vi "Day 4 Task 2.vi"() -> ()   [LabVIEW 2018]
uses:
  <userlib>/_OpenG.lib/array/array.llb/Search 1D Array (I32)__ogtk.vi
  <userlib>/_OpenG.lib/array/array.llb/Conditional Auto-Indexing Tunnel (I32)__ogtk.vi
panel:
  out "all cards won?":bool
  out "final score":i32
  out "number callled":i32
  out "someone won?":bool
  out "card that won":i32
  out "cards":i32[][][](array[numeric])
  out "numbers called out":i32[](array[numeric])
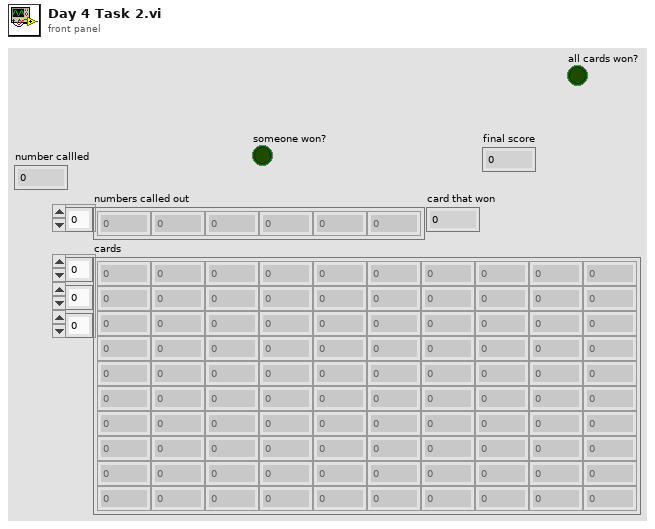
[diagram p1: front panel]
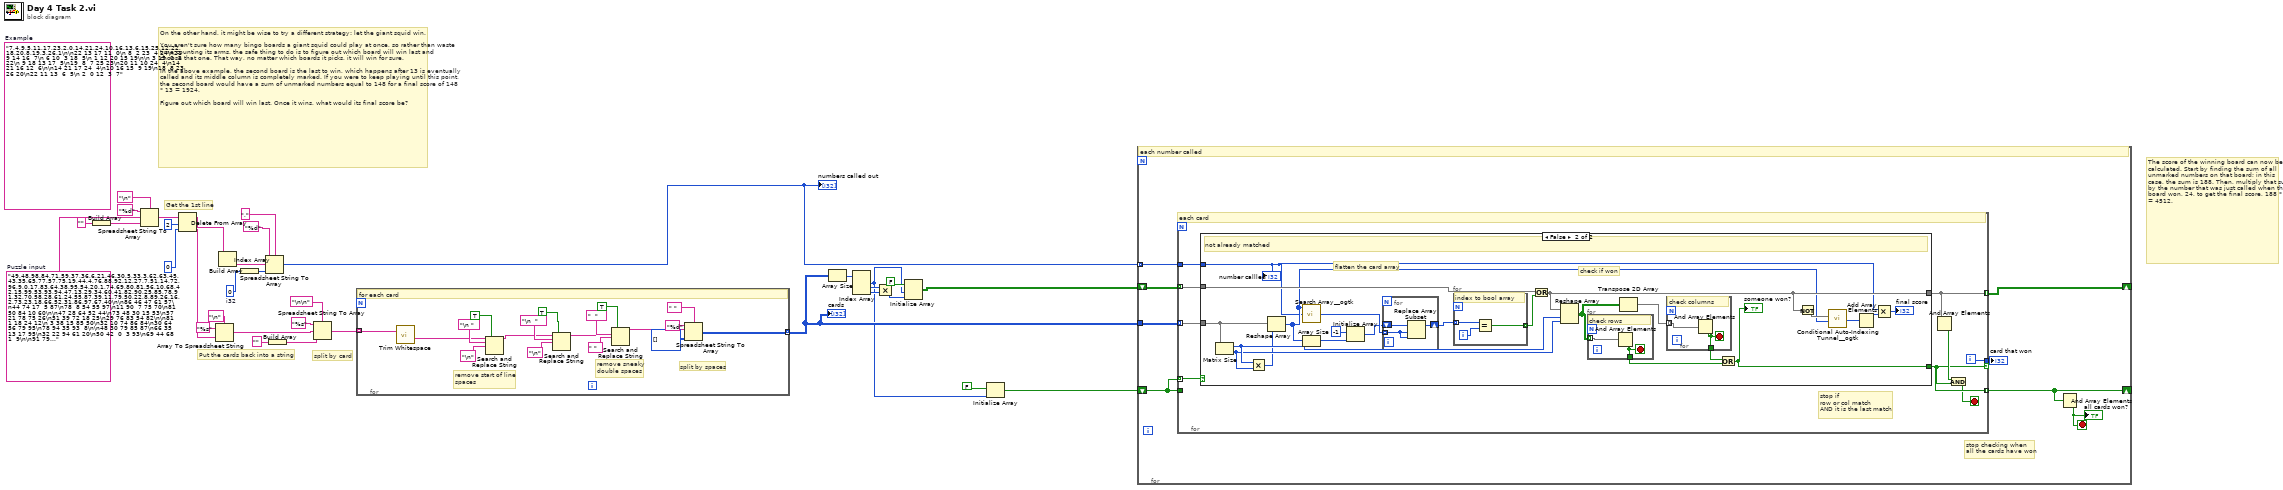
[diagram p0: block diagram]
diagram:
  w1 = "49,48,98,84,71,59,37,36,6,21,46,30,5,33,3,62,63,45,43,35,65,77,57,75,19,44,4,76,88,92,12,27,7,51,14,72,96,9,0,17,83,64,38,95,54,20,1,74,69,80,81,56,10,68,42,15,99,53,93,94,47,13,29,34,60,41,82,90,25,85,78,91,32,70,58,28,61,24,55,87,39,11,79,50,22,8,89,26,16,2,73,23,18,66,52,31,86,97,67,40\n\n86 46 47 61 57\n44 74 17  5 87\n78  8 54 55 97\n11 90  7 75 70\n81 50 84 10 60\n\n47 28 64 52 44\n73 48 30 15 53\n57 21 78 75 26\n51 39 72 18 25\n29 76 83 54 82\n\n81  1 18 24 12\n 3 38 15 85 50\n32 10 74 86 84\n30 64 56 79 95\n78 94 35 93  8\n\n48 30 79 85 87\n66 35 13 17 95\n32 22 94 61 20\n50 42  0  3 93\n69 44 68  1  9\n\n91 79 93 41 33\n98 51 39  9 10\n24 70 99  2 11\n32 13 21  6 68\n40 27 48 89  7\n\n40 29 34  1 23\n79 36 75 57 95\n61 50  4 21 48\n54  0 81 98 72\n24 30 15 31 52\n\n18 68 17 25 34\n97 36 77  6 30\n79 72 38 94 60\n54 45 16 67 12\n58 31 57 71 92\n\n40 58 80 86 85\n91 57 51 23 10\n61 78  4 36 66\n24 41 88 25 99\n15 68 12 55 75\n\n82 99 17  5 76\n65 42 73 78 61\n34 62 14 23 68\n 9 79 72 45  0\n43 96 11 13 10\n\n98 47 90 14 12\n80 63 35 42 11\n27 66  1  9 32\n17 85 61 71 68\n 6 29  7 94 67\n\n38 35 70 18 59\n62 54 84 10 27\n60 92 90 64 86\n25 99 49 43  4\n23 50 39 16 40\n\n72  1 73  8 33\n86 65 99 49 66\n56 79 23 41 46\n 4 48 43 55 93\n98 63 47 37 30\n\n33 96 72 93 99\n30 12 56 46 65\n39 40 59 94 50\n 0  8 67 27 47\n53 57 24 77 42\n\n 9 57  8 28 12\n90 81 21 25 51\n88 18 78  3 64\n20 87 97 45 85\n92 40 52 29 17\n\n99 89 15 54 32\n93 81 36 14 91\n86  7 67 18 92\n65 21 55 38  8\n12 88 27 90 94\n\n96  0  6 91 44\n28 60 10 70 75\n69 37 51 21 87\n93 59 14 53 15\n64 66  9 50 27\n\n33 46 38  2 41\n24 51 50 72 57\n42 85 99 97 56\n35 69 12 86 73\n 4 47 34 80 17\n\n70 28 77 73 53\n67 94 83 79 82\n89  9 96 48 17\n47 86 88 12  3\n55 39 98 14 90\n\n64 82 85 45 10\n27  5 12 72 40\n52 31 25 79 65\n 6 26  3 43 57\n89 49 36 59 35\n\n70  0 58 98 65\n54 93 75 14 26\n28 69 17 29 78\n46 22 47 85 87\n44 38 10 11 63\n\n18 52 66 42 58\n99 78 44 28 73\n24 71  5 14 82\n77 35 45 76 19\n70 20  0 43 48\n\n42 82 85 87 51\n40 49 93 95 74\n25 79 37 67 55\n26 27 90 47 22\n38 50 33 10 75\n\n15 99 60 28 79\n94 42 63 20 57\n44 55 96 67 53\n64  3 29 61 33\n51 12 39 97 30\n\n 7 95 28 39 76\n87 31 23 47 75\n88 10 78 24 20\n30 81 22 51 62\n53 93 55 38  0\n\n12 99  2 89 17\n30 23 92 66 10\n39 60 74 82 15\n 1 28 49  0 29\n90 55  9 69 83\n\n79 44 70 59 88\n90  8 81 23  5\n40 67 66 55 17\n95 61 75 48 91\n98 71 24 38 29\n\n95 28  8 76 13\n86 21 48  3  6\n34 47 31 50  2\n52 40 77 60 61\n 0 88 87 23 25\n\n63 70 34 91 17\n98 49  8  2 14\n25 22 92 65 18\n78 61 97 73 20\n57 83 16  7 68\n\n43 23 70 39 16\n 0 60 76  7 58\n89 40 38 17  5\n86 50 10 77 37\n26 65 25 69 92\n\n34 71 92 19 80\n93  6 24 42 45\n96  9 50 85 21\n36 49 13 25 17\n20 98 74 70 57\n\n25 96 65 77 30\n22 34 41 36 91\n62 18 61 15 19\n42 74 86 58 97\n87 31 53  8 52\n\n40 37 15 53 91\n14 11 35 49 55\n73 32 83 66 87\n98 31 70 58 88\n 7 61  8 76 16\n\n27 94 87 57 80\n54 35 40 59 72\n88 84 70 98 92\n37 52 45  7 16\n 0 30 12 22 41\n\n44 65 68 14 70\n 5 35 17 90  7\n56 89 48 84 32\n73 69 74 51 72\n24 10 94 78 60\n\n81 15  3 42 90\n54 52 74 84 71\n97 78 20  9  2\n59 66  1 91 87\n70 56 93 47 37\n\n93 36 19 69 94\n17 20 48 58 52\n85 57 90 42 14\n16 92  4 49 65\n22  9  2 24 44\n\n47 99 13 31 62\n81 58 88 91 94\n29 11 96 95  1\n14 20 82 34 37\n84 39 76 41 22\n\n 1 74 21  2 67\n38 79 96 26 88\n19 17 94 71 52\n31 28 69  8 51\n41 77 45 95 82\n\n24  9 94 69 65\n97 84 85 53  5\n92 11 61 77  8\n21 75 33 57 63\n43 68 55 52 93\n\n27 21  8 75 73\n 4 53 23 56 47\n28 94 50 80 19\n89 58 24 12 13\n60  5 99 96  9\n\n31 43 59 65 33\n51 32 14 58  4\n11 41 70 78 12\n 1 25 57 80 49\n91 66  0 27 17\n\n64 67 37 24 35\n 4 22 54 75 21\n19 91  9 52 83\n20 68 53 12  0\n28 76 51 49 89\n\n67 89 14 54 81\n 0 59 51 63 56\n85 88 95  7 36\n40 27 47 86 19\n52 92 22 16 30\n\n75 25 39  9 19\n59 92 24  6 22\n79 73 34 66 49\n16 89 56 76 55\n 5 45  4 46 62\n\n71 44 63 97 47\n27 61 70 52 46\n19 80 21 68 65\n28 45 84 14 94\n38 73 66 78 92\n\n47 45 41 96 54\n38 14 62 55 91\n 2 11 97 12 51\n36 49  3 95 76\n 5 75  7 94 87\n\n70 24 93 96 86\n49 51 73 50 83\n97  0 57 13  9\n99 46 22 67 39\n56 21 29 52 27\n\n42 82 80 65 19\n78 41 56 83 75\n51 72 10  1 33\n84 63 21 87 86\n77 64 31 68  6\n\n60 50 31  5 58\n83  9 87 98 13\n 4 35 24 33 88\n54 59 71 64  3\n16 57 48 15 86\n\n45 29 81 25 14\n13 21 79 90  0\n88 38 56 11 15\n47  2 40 35 75\n91 28 48 32 98\n\n87 58 78 65 69\n89 35 45 26 13\n28 61 15  3 44\n64 57 92 93 50\n90 39  4 70  9\n\n16 35 41 40 81\n48 92 94 83 79\n54 50 62  8 53\n14  5 85 68 22\n42 26 33 23 93\n\n 7 13 82 89 49\n43 21 79 38 56\n 6 31 90 58 81\n39 47 77 30 54\n23 41 86 19  8\n\n69 20 95 33 63\n64 34  4 79 36\n13 21 78 56  6\n35 44 85 27 76\n75 15 14 52 39\n\n42 71 73  1 45\n66 75  7 40 54\n91 83 65 53 20\n34 97 88  5 61\n63 82 50 74 38\n\n62 89 40 70 91\n84 12 19 96 79\n72 15 35 23 14\n 4 69  0 55 17\n85 90 20 28 13\n\n27 93 23  1 38\n67 28 62  9 96\n31 35 47 44 88\n78 57 53  5 69\n91 15 82 75 61\n\n17 44 85 92 94\n 0 67  5 50 64\n66 65 98 58 56\n62  4 57 99 34\n83 43 76 12 69\n\n 0 28 13 68 86\n84 24 50 32 40\n25 71 72 96 94\n89  1 64 81 23\n97 66  5 15 91\n\n59 67 79 84 44\n74 61 81 20 68\n24 92 55 99 11\n76 60 97 43 66\n31 30 89 45 53\n\n 1 97 15 34 85\n45 59 54 66 24\n53 36 51 58 27\n84 83 71  5 95\n70  6 65 79 13\n\n84 86  0 25  2\n 1 59 92 39 56\n17  7 88 78 24\n51 87 89 44 31\n54 63 50 18 36\n\n98 86 30 70 12\n11 52 49 39 14\n16 35 56 87 72\n85 65 93 92 60\n20 43 77 41 79\n\n50 31 71 78 21\n70 94 99 35 29\n56 58 27 65 28\n45 36 47 69 98\n 5 48 61 19 93\n\n64 65 86 14 53\n 7 43 75 39 38\n20 59 80 88 54\n12 32 66 34 87\n29 15 25 19 45\n\n88 20 42  5 32\n56  8 80 15 98\n36 99 35 27 16\n92 66 75 91 10\n81 96 65  0 57\n\n29 78  8 76 41\n99 18 60 90 47\n50 51 40  2 31\n38 70 25 52 39\n26 35 84  6 80\n\n 6 68 56 15 53\n99 60 69 25  7\n65 35  9 11 66\n92 85 48 40 97\n63 59 57 17 55\n\n46 95 75 99 21\n50 24 64 35 63\n93 39  3 67 82\n41 42 84 15 55\n79 81 97 60 17\n\n33 14 60 42 40\n76 73 56 71 88\n91 41 83 74 16\n57 85 35 44 47\n99 59 46 12 45\n\n53 83 54 21 68\n79 97 85  0 67\n41 90 48 95  3\n96 70 65 22 25\n60 77 33 15 28\n\n17 12  5 51 15\n75 92 72 16 65\n59 85 29 23 57\n14 53 97 68 84\n 1 93 49 38 28\n\n27 40 24 12 57\n84 13  9 43 31\n70 23 51 94 34\n 1 80 91 16 29\n99 75 49 52 54\n\n52 85 23 72 40\n 6 88 16 41 67\n53 94  8 32 33\n75 62 24 13 64\n65  0 60 86 47\n\n 5 28 27 15 41\n19 77 38 83 45\n32 70 78 26 90\n82 80 85 22 84\n59 73 24  9 63\n\n29 58 28 82 13\n78 55 63 43 51\n19 33 90 91 48\n93  7 35 22 71\n40 95 38 24 46\n\n38 30 13 16 74\n69 68 42  6  4\n62 82 29 79  1\n61  7 15 25 85\n 5 66 45 43 90\n\n19 65 12 91 34\n17  6 30 32 64\n37 53  4 35 62\n41 22 13 11 25\n60 27 93 76 51\n\n 3 92 25 88 14\n40 30 55 10 37\n19 94 56 34 74\n75 87 80 54 83\n 2 20 70 45 16\n\n52 93 87 60 11\n82 66 88 59 95\n58 31 49 33 28\n77 39 43  9 51\n20 80 98 47 16\n\n35 48 47 11 82\n 8 36 54 20 40\n90 95 85  4 66\n22 75 64 81 10\n27 62 89 30 12\n\n75 40 11 63 19\n 4 43  6 93 48\n85 58 82 66 52\n32 28  0 14 20\n78 61 83 95 87\n\n57 79 16 37 33\n20 17 27 38 63\n35 77 60 97 34\n22 78 72 43 26\n29 12  9 46 54\n\n26 94 37 57  1\n49  6 65 80 55\n46 38 33 89 99\n42 18 86 97 98\n45 76 41  9 12\n\n83 70 31 61 30\n16 78 84 12 18\n15 65 62 55 98\n 6 21 80 41 69\n25  2 24 10 79\n\n98 75  5 66 37\n90  7 26 61 15\n48 70 20 60 41\n23 58 82 22 74\n80  8 51 67 55\n\n84 86 77 97 28\n37 87  2 93  5\n16 64 35 61 27\n 8  3 36 10 73\n31 65 94 63 13\n\n91  9 64 67 19\n56 35 11 62 28\n 0 65 59 72 45\n34 24 51 26 80\n93 50 58 53 27\n\n27 54 77 57 94\n60 46 55 74 62\n16  9 19 48  6\n69  1 26 78  2\n45 75 41 25 90\n\n45 83 97 81 95\n26 64 40 94  7\n57 28 86  8 36\n98 92 16 13 20\n99 79 50 65 51\n\n38  6 96 71 10\n51 55  2 44 74\n31 61 98 72 73\n79 54 91 34 62\n88 17 46 45 43\n\n17 18 39 59 26\n45 40 91 47 74\n46 97 94 12 79\n61  7  8 56 50\n 0 77 20 57  9\n\n74  4 65  2 23\n45 56 90 94 96\n80 71 69 86 85\n19 78 35 47 98\n51 73  6 33 14\n\n 8 60 40  2 37\n10 68 44 50 73\n69 26  6 52 93\n33 65 46 24 11\n71 59 15 28 84\n\n57 65 70 98 68\n80  3 13 39 20\n11 71 47 78 42\n31 61 72 86  9\n53 43 87 28 77\n\n67 32 59 34 77\n29 23 80 27 62\n81 97 46 14 42\n19 47 44 85 24\n53  9 71 37  1\n\n83 13 27 41  9\n95 62 65 86 63\n 0 17 33 11 76\n45 64 39 71 55\n84 52 21 59 20\n\n63 45 55 80  3\n14 73 47 96 10\n82 26 85  0 11\n53  6 28 57 60\n49 99 18 50 71\n\n30 67 16 22 84\n81  4 34 61 65\n57 69 51 94 58\n 6 89 37 75 47\n19 14 97  2 86\n\n64 83  1 66 70\n30 82 96  3 67\n79 11 22 95 14\n87 60  4 15 26\n84 69 99 19 74"  # Puzzle input
  w13 = 0  # i32
  (unwired) "7,4,9,5,11,17,23,2,0,14,21,24,10,16,13,6,15,25,12,22,18,20,8,19,3,26,1\n\n22 13 17 11  0\n 8  2 23  4 24\n21  9 14 16  7\n 6 10  3 18  5\n 1 12 20 15 19\n\n 3 15  0  2 22\n 9 18 13 17  5\n19  8  7 25 23\n20 11 10 24  4\n14 21 16 12  6\n\n14 21 17 24  4\n10 16 15  9 19\n18  8 23 26 20\n22 11 13  6  5\n 2  0 12  3  7"  # Example
  # "On the other hand, it might be wise to try a different strategy: let the giant squid win.\n\nYou aren't sure how many bingo boards a giant squid could play at once, so rather than waste time counting its arms, the safe thing to do is to figure out which board will win last and choose that one. That way, no matter which boards it picks, it will win for sure.\n\nIn the above example, the second board is the last to win, which happens after 13 is eventually called and its middle column is completely marked. If you were to keep playing until this point, the second board would have a sum of unmarked numbers equal to 148 for a final score of 148 * 13 = 1924.\n\nFigure out which board will win last. Once it wins, what would its final score be?"
  # "The score of the winning board can now be calculated. Start by finding the sum of all unmarked numbers on that board; in this case, the sum is 188. Then, multiply that sum by the number that was just called when the board won, 24, to get the final score, 188 * 24 = 4512."
  # "split by card"
  # "Put the cards back into a string"
  # "Get the 1st line"
  n1 = Build Array("") -> (w31:string[])
  n2 = Spreadsheet String To Array(delimiter (Tab)="\n", format string="%d", spreadsheet string=w1, array type (2D Dbl)=w31) -> (array=w29:string[])
  n3 = Delete From Array(array=w29, length=2, index=0) -> (deleted portion=w24:string[], array with subset deleted=w21:string[])
  n4 = Array To Spreadsheet String(delimiter (Tab)="\n", array=w21, 3:"%s" ("format string")) -> (spreadsheet string=w19:string)
  n5 = Index Array(array=w24) -> (element=w15:string)  [unwired: 1 in]
  n6 = Build Array(w13) -> (w14:i32[])
  n7 = Spreadsheet String To Array(delimiter (Tab)=",", format string="%d", spreadsheet string=w15, array type (2D Dbl)=w14) -> (array=w11:i32[])
  "numbers called out" <- w11
  n8 = Build Array("") -> (w16:string[])
  n9 = Spreadsheet String To Array(delimiter (Tab)="\n\n", format string="%s", spreadsheet string=w19, array type (2D Dbl)=w16) -> (array=w18:string[])
  n10 = for {
    tunnel: w18 -> [w35] mode=indexing
    tunnel: [w48] -> w10 mode=indexing
    # "remove start of line\nspaces"
    # "split by spaces"
    # "remove sneaky\ndouble spaces"
    # "for each card"
    n11 = call <vilib>:"Trim Whitespace.vi"("string"=w35) -> ("trimmed string"=w34:string)  [unwired: 1 in]
    n12 = Search and Replace String(replace all?=TRUE ("replace all? (F)"), input string=w34, search string="\n " ("delimiter (Tab)"), replace string="\n" ("delimiter (Tab)")) -> (result string=w38:string)  [unwired: 4 in, 3 out]
    n13 = Search and Replace String(replace all?=TRUE ("replace all? (F)"), input string=w38, search string="\n  " ("delimiter (Tab)"), replace string="\n" ("delimiter (Tab)")) -> (result string=w37:string)  [unwired: 4 in, 3 out]
    n14 = Search and Replace String(replace all?=TRUE ("replace all? (F)"), input string=w37, search string="  " ("delimiter (Tab)"), replace string=" " ("delimiter (Tab)")) -> (result string=w44:string)  [unwired: 4 in, 3 out]
    n15 = Spreadsheet String To Array(delimiter (Tab)=" ", format string="%d", spreadsheet string=w44, array type (2D Dbl)=i32[][] []) -> (array=w48:i32[][])
  }
  "cards" <- w10
  n16 = Array Size(array=w10) -> (size(s)=w9:i32[])
  n17 = Index Array(array=w9) -> (element #1=w3:i32, element #3=w6:i32)  [unwired: 3 in, 1 out]
  n18 = Multiply(x=w6, y=w6) -> (x*y=w5:i32)
  n19 = Initialize Array(FALSE, w3, w5) -> (w7:bool[][])
  n20 = Initialize Array(FALSE, w3) -> (w2:bool[])
  n21 = for {
    tunnel: w10 -> [w59]
    tunnel: w11 -> [w58] mode=indexing
    shift-right: [w56] -> _
    shift-left: w7 -> [w57]
    shift-right: [w53] -> _
    shift-left: w2 -> [w52]
    stop <- w54 stop-if-true
    # "stop checking when\nall the cards have won"
    # "each number called"
    n22 = for {
      tunnel: w59 -> [w68] mode=indexing
      tunnel: w58 -> [w66]
      tunnel: w57 -> [w67] mode=indexing
      tunnel: [w64] -> w56 mode=indexing
      tunnel: [w63] -> w55 if=w61
      tunnel: w52 -> [_]
      tunnel: [w61] -> w53 mode=indexing
      tunnel: w52 -> [w65] mode=indexing
      i -> [w63]
      stop <- w60 stop-if-true
      # "stop if\nrow or col match\nAND it is the last match"
      # "each card"
      n23 = case shown="False" w65 {
        selector: w65 -> [w69 _]
        tunnel: w68 -> [_ w93]
        tunnel: w67 -> [w70 w91]
        tunnel: [w70 w78] -> w64
        tunnel: w66 -> [_ w73]
        tunnel: [w69 w71] -> w61
        frame True {
          # "This card already won"
        }
        frame False {
          # "check if won"
          # "flatten the card array"
          # "not already matched"
          n24 = Matrix Size(0:w93) -> (1:w86:i32, 2:w85:i32)
          n25 = Multiply(x=w86, y=w85) -> (x*y=w84:i32)
          n26 = Reshape Array(w93, w84) -> (w76:i32[])
          n27 = call-poly <userlib>:"Search Array__ogtk.vi"("Array"=w76, "Element Data"=w73) -> ("Indices of Elements"=w80:i32[])  [unwired: 7 in]
          n28 = Array Size(array=w76) -> (size(s)=w82:i32)
          n29 = Initialize Array(-1 ("Numeric"), w82) -> (w79:i32[])
          n30 = for {
            tunnel: w80 -> [w103] mode=indexing
            shift-right: [w102] -> w81
            shift-left: w79 -> [w101]
            n31 = Replace Array Subset(array=w101, new element=w103, index=w103) -> (w102:i32[])
          }
          n32 = for {
            tunnel: [w100] -> w92 mode=indexing
            tunnel: w81 -> [w98] mode=indexing
            i -> [w99]
            # "index to bool array"
            n33 = Equal?(x=w98, y=w99) -> (x = y?=w100:bool)
          }
          n34 = Or(x=w91, y=w92) -> (x .or. y?=w78:bool[])
          n35 = Reshape Array(w78, w86, w85) -> (w90:bool[][])
          n36 = for {
            tunnel: w90 -> [w97] mode=indexing
            tunnel: [w96] -> w87
            stop <- w96 stop-if-true
            # "check rows"
            n37 = And Array Elements(Boolean array=w97) -> (logical AND=w96:bool)
          }
          n38 = Transpose 2D Array(2D array=w90) -> (transposed array=w89:bool[][])
          n39 = for {
            tunnel: w89 -> [w95] mode=indexing
            tunnel: [w94] -> w88
            stop <- w94 stop-if-true
            # "check columns"
            n40 = And Array Elements(Boolean array=w95) -> (logical AND=w94:bool)
          }
          n41 = Or(x=w88, y=w87) -> (x .or. y?=w71:bool)
          "someone won?" <- w71
          n42 = Not(x=w78) -> (.not. x?=w77:bool[])
          n43 = call-poly <userlib>:"Conditional Auto-Indexing Tunnel__ogtk.vi"("Array in"=w76, "Elements to keep"=w77) -> ("Filtered Array out"=w75:i32[])  [unwired: 5 in]
          n44 = Add Array Elements(numeric array=w75) -> (sum=w74:i32)
          n45 = Multiply(x=w73, y=w74) -> (x*y=→"final score":i32)
          "number callled" <- w73
        }
      }
      n46 = And Array Elements(Boolean array=w64) -> (logical AND=w62:bool)
      n47 = And(x=w62, y=w61) -> (x .and. y?=w60:bool)
    }
    "card that won" <- w55
    n48 = And Array Elements(Boolean array=w53) -> (logical AND=w54:bool)
    "all cards won?" <- w54
  }
